vi "1D Kalman Filter Accelerometer - Final (lite).vi"(10 "Step Size (s)":dbl, 11 "Error":errorcluster) -> (0 "Acceleration (cm/s^2)":dbl, 1 "Speed (cm/s)":dbl, 2 "Displacement (cm)":dbl, 3 "Error out":errorcluster, 4 "State":enum16{"Braking", "Coast", "Accelerating"}(ring))   [LabVIEW 2017]
doc: "This VI demonstrate how to use the Continuous Kalman Filter to track the location of a 'robot' \nbased on three different situations:\n\n 1 - Only using the Encoder Measurement\n 2 - Only using the Accelerometer Measurement\n 3 - Using Encoder and Accelerometer"
uses:
  <vilib>/addons/Control Design/_Stochastic Systems/NI_CD_Stochastic Systems.lvlib
  <vilib>/addons/Control Design/_Stochastic Systems/Stochastic Systems.llb/CD Construct Stochastic Model (Numeric).vi
  <vilib>/Simulation/Scripting/Companion Diagram/SimConfigNode/SimDog.xnode
  <vilib>/Simulation/Scripting/Companion Diagram/SimConfigNode/SimParams.ctl
  <vilib>/Simulation/Implementation/Shared/SIMSCR Execution Mode.ctl
  <vilib>/Simulation/Scripting/Companion Diagram/SimConfigNode/_simSolvers.ctl
  <vilib>/Simulation/Implementation/XNodeFramework/SimXNode/SimX.xnode
  <vilib>/addons/Control Design/_Implementation/CD Continuous Recursive Kalman Filter.vi
  <vilib>/Simulation/Utility/Implementation/SIM Halt.vi
  National Instruments/LabVIEW 2017/examples/Control and Simulation/Algorithms/Kalman Filter/subVIs/1D Kalman - Update Measurement Noise.vi
  <vilib>/myRIO/Express VI/Onboard Devices/Accelerometer/Accelerometer Express VI.xnode
  <vilib>/addons/Control Design/_Stochastic Systems/Stochastic Systems.llb/CD Construct Noise Model (Numeric).vi
  <vilib>/myRIO/Instrument Drivers/Onboard Devices/Accelerometer/vis/Read.vi
  <vilib>/myRIO/Instrument Drivers/Onboard Devices/Accelerometer/Accelerometer.lvlib
  <vilib>/myRIO/Common/Instrument Driver Framework/myRIO v1.0/Accelerometer/typedefs/Accelerometer Channels Enum.ctl
  <vilib>/myRIO/Common/Instrument Driver Framework/myRIO v1.0/Accelerometer/typedefs/Accelerometer Channels List.ctl
  <vilib>/myRIO/Common/Instrument Driver Framework/Utilities/typedefs/Generic FPGA Reference.ctl
  <vilib>/myRIO/Common/Instrument Driver Framework/Utilities/typedefs/myRIO v1.0 Reference.ctl
  <vilib>/myRIO/Common/Instrument Driver Framework/Utilities/typedefs/Hardware Version Enum.ctl
  <vilib>/myRIO/Common/Instrument Driver Framework/Utilities/typedefs/myRIO Generic Hardware Reference.ctl
  <vilib>/myRIO/Instrument Drivers/Onboard Devices/Accelerometer/typedefs/Accelerometer Reference.ctl
  <vilib>/myRIO/Instrument Drivers/Onboard Devices/Accelerometer/vis/myRIO Accelerometer Open.xnode
  <vilib>/myRIO/Common/Instrument Driver Framework/Utilities/vis/Is FPGA Ref Available.vi
  <vilib>/ptbypt/Probability & Statistics.llb/Mean PtByPt.vi
  <vilib>/ptbypt/NI_PtbyPt.lvlib
  <vilib>/myRIO/Common/Instrument Driver Framework/myRIO v1.0/Accelerometer/vis/myRIO v1.1 Open Accelerometer.vi
  <vilib>/userdefined/High Color/nirio_resource_hc.ctl
  <vilib>/Simulation/Implementation/Shared/SIM Bundle Sim Info.vi
  <vilib>/Simulation/Implementation/Shared/SIM Unbundle Sim Info.vi
  <vilib>/Simulation/Implementation/Shared/NILVSim_FinalizeModel.vi
  <vilib>/Simulation/Implementation/Shared/NILVSim_GetModelError.vi
  <vilib>/Platform/TimedLoop/XDataNode/wakeup.ctl
  <vilib>/Platform/TimedLoop/XDataNode/XDNodeRunTimeDep.lvlib
  <vilib>/Platform/TimedLoop/XDataNode/nitl_modes.ctl
  <vilib>/Platform/TimedLoop/XDataNode/timing_clust.ctl
  <vilib>/platform/TimedLoop/XDataNode/XDataNode.xnode
  <vilib>/Simulation/Implementation/Shared/NILVSim_Initialize.vi
  <vilib>/Simulation/Implementation/Shared/NILVSim_FinishedLate.vi
  <vilib>/Simulation/Utility/Implementation/NILVSim Get Time and IsAcceptedStep.vi
  <vilib>/Simulation/Implementation/Shared/NILVSim_Manager.vi
  <vilib>/Simulation/Implementation/Shared/NI_SIM_Implementation.lvlib
  <vilib>/Simulation/Implementation/Shared/NILVSIM_BeginStep.vi
  <vilib>/Simulation/Param Hierarchy/Typedefs/SIMPH Param Control Actions.ctl
  <vilib>/Simulation/Implementation/Shared/NILVSim_ParamChanged.vi
  <vilib>/Utility/error.llb/Clear Errors.vi
  <vilib>/Simulation/Implementation/Shared/SIMSH Read Queue.vi
  <vilib>/addons/Control Design/_Stochastic Systems/Stochastic Systems.llb/Stochastic Systems SubVIs/cd_Second-Order Statistics Noise Model.ctl
  <vilib>/Simulation/Implementation/Shared/SIM Is Init or Final Stage.vi
panel:
  out "Filtered Mean (g)":dbl format="%0.2f"
  in  "Accelerometer Bias\ncm/s^2":dbl
  in  "Halt?":bool
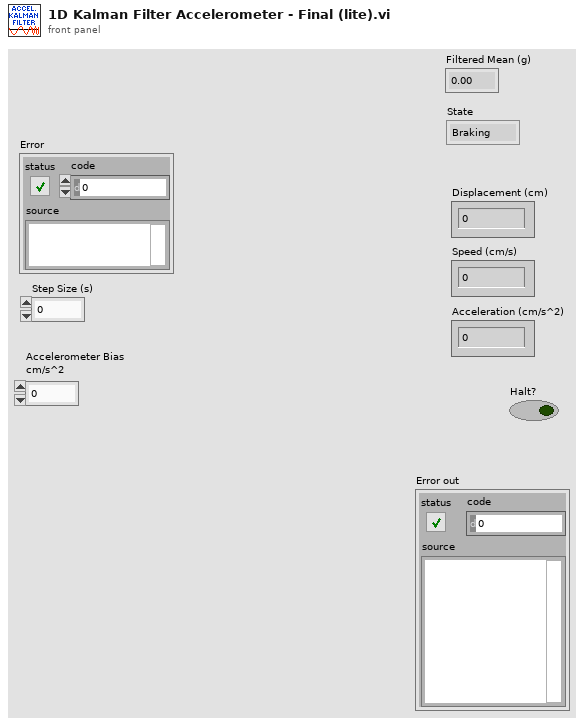
[diagram p1: front panel]
types:
  T1 = typedef "NI_CD_Stochastic Systems.lvlib/cd_Stochastic State-Space Model.ctl" = cluster{"Sampling Time (s)":dbl, "G":dbl[][], "B":dbl[][], "A":dbl[][], "C":dbl[][], "D":dbl[][], "H":dbl[][]}
  T2 = typedef "NI_CD_Stochastic Systems.lvlib/cd_Second-Order Statistics Noise Model.ctl" = cluster{"Q":dbl[][], "E{w}":dbl[], "E{v}":dbl[], "R":dbl[][], "N":dbl[][]}
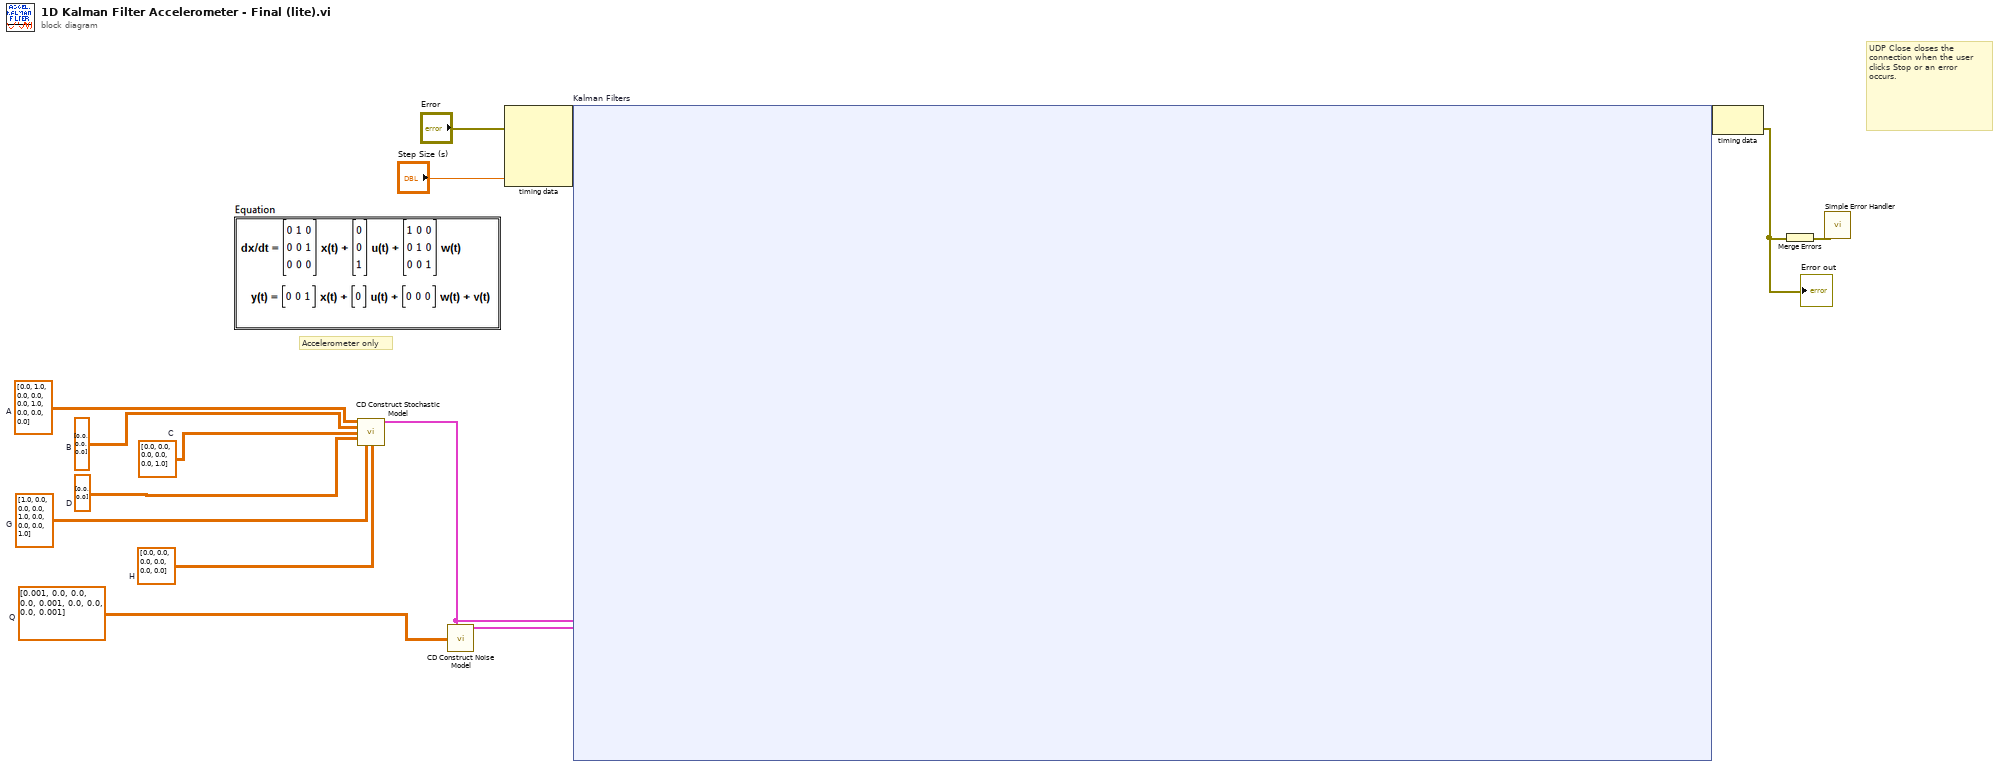
[diagram p0: block diagram]
diagram:
  w4 = dbl[][] [[0.0, 0.0, 0.0], [0.0, 0.0, 1.0]]  # C
  w9 = dbl[][] [[0.0], [0.0]]  # D
  w8 = dbl[][] [[0.001, 0.0, 0.0], [0.0, 0.001, 0.0], [0.0, 0.0, 0.001]]  # Q
  w7 = dbl[][] [[0.0, 0.0, 0.0], [0.0, 0.0, 0.0]]  # H
  w6 = dbl[][] [[1.0, 0.0, 0.0], [0.0, 1.0, 0.0], [0.0, 0.0, 1.0]]  # G
  w5 = dbl[][] [[0.0], [0.0], [0.0]]  # B
  w10 = dbl[][] [[0.0, 1.0, 0.0], [0.0, 0.0, 1.0], [0.0, 0.0, 0.0]]  # A
  # "UDP Close closes the connection when the user clicks Stop or an error occurs."
  # "Accelerometer only"
  n1 = call-poly <vilib>:"CD Construct Stochastic Model.vi"("A"=w10, "B"=w5, "C"=w4, "D"=w9, "G"=w6, "H"=w7) -> ("Stochastic State-Space Model"=w12:T1)  [unwired: 8 in, 1 out]
  n2 = call-poly <vilib>:"CD Construct Noise Model.vi"("Stochastic State-Space Model"=w12, "Q"=w8) -> ("Second-Order Statistics Noise Model out"=w13:T2)  [unwired: 12 in, 1 out]
  n3 = node-c288("Error", "Step Size (s)") -> (w15:variant)  [unwired: 3 in]
  n4 = node-c254 "Kalman Filters"(w15, w13, w12) -> (w14:variant)
  n5 = node-c288(w14) -> (w1:errorcluster)
  "Error out" <- w1
  n6 = Merge Errors(w1) -> (w11:errorcluster)
  n7 = call <vilib>:"Simple Error Handler.vi"("error in (no error)"=w11) -> ()  [unwired: 4 in, 5 out]
